vi "Build Tree.vi"(5 "Defer Updates (T)":bool=TRUE, 7 "Tree":refnum<vi>, 8 "error in":errorcluster, 11 "Tree Map in":refnum<class "Project Tree Map.lvclass">) -> (0 "error out":errorcluster, 3 "Tree Map out":refnum<class "Project Tree Map.lvclass">)   [LabVIEW 2020, in "VI Properties Editor.lvlib" / "Project Tree Map.lvclass"]
doc: "Builds the tree by adding the tree items one at a time."
uses:
  Project Tree Map.lvclass
  Project Tree Map.lvclass/Project Tree Map.ctl
  VI Properties Editor.lvlib
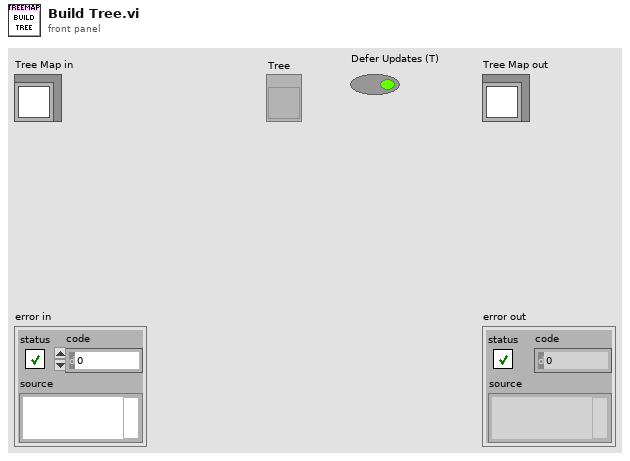
[diagram p1: front panel]
types:
  T1 = typedef "LVNodeAndColumnTypeDef.ctl" = cluster{"Node":string, "Column":i32}
  T2 = typedef "VI Properties Editor.lvlib/Project Tree Map.lvclass/Tree Key.ctl" = cluster{"Order":i32, "Hierarchy":string[]}
  T3 = typedef "VI Properties Editor.lvlib/Project Tree Map.lvclass/Tree Entry.ctl" = cluster{"Hierarchy":string[], "Name":string, "Columns":string[], "BG Color":u32, "Leaf":bool, "Symbol":string, "Parent Tag":string, "Order":i32, "Tag":string}
  T4 = typedef "imagedata.ctl" = cluster{"image type":i32, "image depth":i32, "image":u8[], "mask":u8[], "colors":u32[], "Rectangle":cluster{"left":i16, "top":i16, "right":i16, "bottom":i16}}
  T5 = map{string, cluster{"index":i32, "image data":T4}}
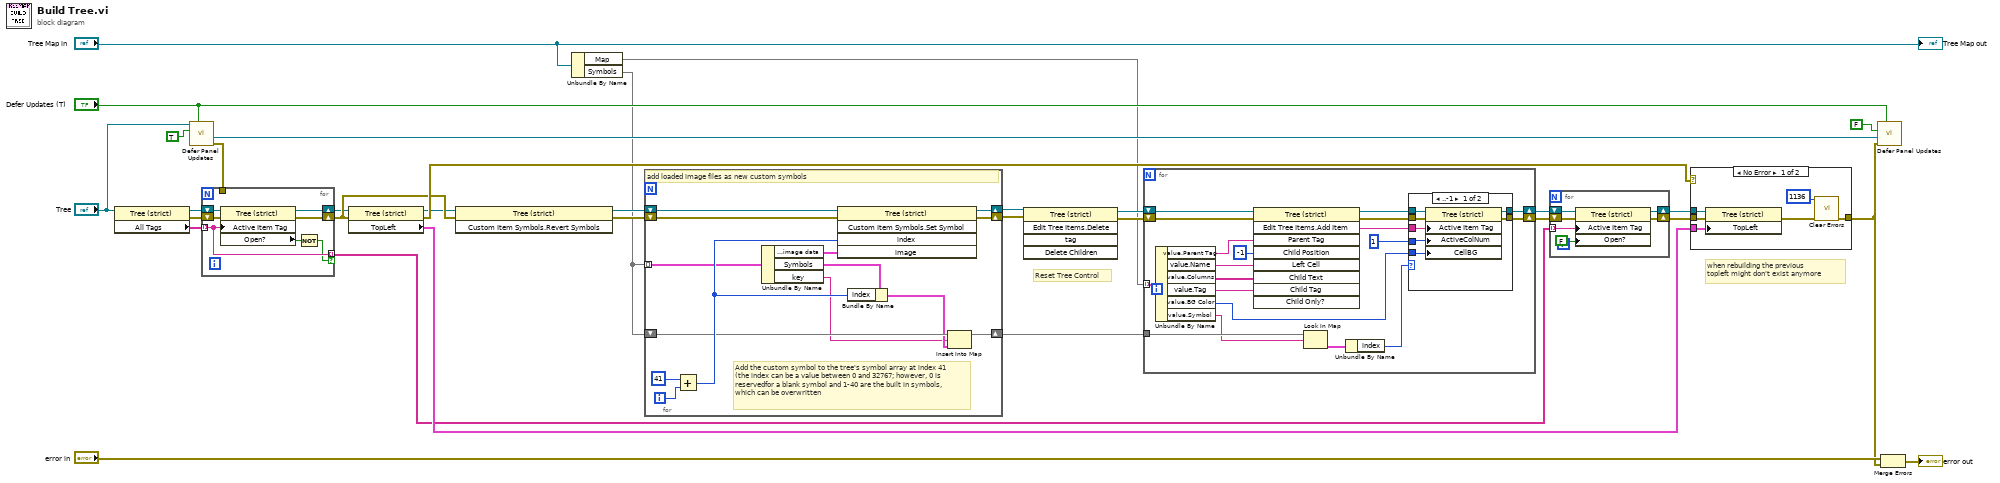
[diagram p0: block diagram]
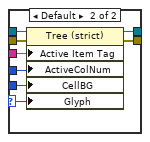
[diagram p2: hidden frame]
diagram:
  # "when rebuilding the previous\ntopleft might don't exist anymore"
  # "Reset Tree Control"
  n1 = property on="Property Node" class="Tree (strict)"(reference="Tree") -> (reference out=w17:refnum<vi>, error out=w29:errorcluster, "All Tags"=w18:string[])  [unwired: 1 in]
  n2 = call "Defer Panel Updates.vi"("Set Defer (T)"="Defer Updates (T)", "Defer"=TRUE, "Tree (Front Panel)"="Tree") -> ("error out"=w30:errorcluster, "Front Panel"=w9:refnum<vi>)  [unwired: 7 in]
  n3 = for {
    tunnel: w18 -> [w35] mode=indexing
    shift-right: [w33] -> w16
    shift-left: w17 -> [w37]
    tunnel: [w35] -> w15 mode=indexing if=w34
    tunnel: w30 -> [_]
    shift-right: [w38] -> w22
    shift-left: w29 -> [w39]
    n4 = property on="Property Node" class="Tree (strict)"(reference=w37, error in=w39, "Active Item Tag"=w35) -> (reference out=w33:refnum<vi>, error out=w38:errorcluster, "Open?"=w36:bool)
    n5 = Not(x=w36) -> (.not. x?=w34:bool)
  }
  n6 = property on="Property Node" class="Tree (strict)"(reference=w16, error in=w22) -> (reference out=w5:refnum<vi>, error out=w24:errorcluster, "TopLeft"=w19:T1)
  n7 = invoke on="Invoke Node" class="Tree (strict)" method="Custom Item Symbols.Revert Symbols"(reference=w5, error in=w22) -> (reference out=w4:refnum<vi>, error out=w23:errorcluster)  [unwired: 1 in, 1 out]
  n8 = Unbundle By Name("Tree Map in") -> ("Map"=w6:map{T2, T3}, "Symbols"=w3:T5)
  n9 = for {
    shift-right: [w49] -> w1
    shift-left: w4 -> [w50]
    shift-right: [w51] -> w21
    shift-left: w23 -> [w52]
    tunnel: w3 -> [w45] mode=indexing
    shift-right: [w43] -> w2
    shift-left: w3 -> [w44]
    i -> [w48]
    # "Add the custom symbol to the tree's symbol array at index 41 (the index can be a value between 0 and 32767; however, 0 is reservedfor a blank symbol and 1-40 are the built in symbols, which can be overwritten"
    # "add loaded image files as new custom symbols"
    n10 = Add(x=41 ("Index"), y=w48) -> (x+y=w53:i32)
    n11 = Unbundle By Name(w45) -> ("Symbols.image data"=w47:T4, "Symbols"=w41:cluster{"index":i32, "image data":T4}, "key"=w40:string)
    n12 = invoke on="Invoke Node" class="Tree (strict)" method="Custom Item Symbols.Set Symbol"(reference=w50, error in=w52, "index"=w53, "image"=w47) -> (reference out=w49:refnum<vi>, error out=w51:errorcluster)  [unwired: 1 in, 3 out]
    n13 = Bundle By Name(cluster=w41, "index"=w53) -> (w42:cluster{"index":i32, "image data":T4})
    n14 = Insert Into Map(map in=w44, key=w40, value=w42) -> (map out=w43:T5)  [unwired: 2 out]
  }
  n15 = invoke on="Invoke Node" class="Tree (strict)" method="Edit Tree Items.Delete"(reference=w1, error in=w21) -> (reference out=w20:refnum<vi>, error out=w32:errorcluster)  [unwired: 3 in, 3 out]
  n16 = for {
    shift-right: [w66] -> w13
    shift-left: w20 -> [w70]
    tunnel: w6 -> [w67] mode=indexing
    shift-right: [w71] -> w28
    shift-left: w32 -> [w72]
    tunnel: w2 -> [w65]
    n17 = Unbundle By Name(w67) -> ("value.Parent Tag"=w63:string, "value.Name"=w68:string, "value.Columns"=w69:string[], "value.Tag"=w62:string, "value.BG Color"=w64:u32, "value.Symbol"=w61:string)
    n18 = invoke on="Invoke Node" class="Tree (strict)" method="Edit Tree Items.Add Item"(reference=w70, error in=w72, "Parent Tag"=w63, "Child Position"=-1, "Left Cell"=w68, "Child Text"=w69, "Child Tag"=w62) -> (reference out=w59:refnum<vi>, error out=w60:errorcluster, "Edit Tree Items:Add Item"=w58:string)  [unwired: 2 in, 6 out]
    n19 = Look In Map(map=w65, key=w61) -> (value=w56:cluster{"index":i32, "image data":T4})  [unwired: 1 in, 1 out]
    n20 = Unbundle By Name(w56) -> ("index"=w55:i32)
    n21 = case shown="..-1" w55 {
      selector: w55 -> [_ w80]
      tunnel: w59 -> [w77 w85]
      tunnel: w60 -> [w79 w87]
      tunnel: w58 -> [w73 w84]
      tunnel: 1 ("Active Cell:Active Column Number") -> [w74 w83]
      tunnel: [w76 w82] -> w66
      tunnel: [w78 w86] -> w71
      tunnel: w64 -> [w75 w81]
      frame ..-1 {
        n22 = property on="Property Node" class="Tree (strict)"(reference=w77, error in=w79, "Active Item Tag"=w73, "ActiveColNum"=w74, "CellBG"=w75) -> (reference out=w76:refnum<vi>, error out=w78:errorcluster)
      }
      frame Default {
        n23 = property on="Property Node" class="Tree (strict)"(reference=w85, error in=w87, "Active Item Tag"=w84, "ActiveColNum"=w83, "CellBG"=w81, "Glyph"=w80) -> (reference out=w82:refnum<vi>, error out=w86:errorcluster)
      }
    }
  }
  n24 = for {
    shift-right: [w90] -> w14
    shift-left: w13 -> [w91]
    tunnel: w15 -> [w88] mode=indexing
    shift-right: [w92] -> w27
    shift-left: w28 -> [w93]
    n25 = property on="Property Node" class="Tree (strict)"(reference=w91, error in=w93, "Active Item Tag"=w88, "Open?"=FALSE ("Active Item:Open?")) -> (reference out=w90:refnum<vi>, error out=w92:errorcluster)
  }
  n26 = case shown="No Error" w24 {
    tunnel: w19 -> [w96 _]
    tunnel: w14 -> [w95 _]
    tunnel: w27 -> [w99 w100]
    tunnel: [w97 w100] -> w25
    frame No Error {
      n27 = property on="Property Node" class="Tree (strict)"(reference=w95, error in=w99, "TopLeft"=w96) -> (error out=w98:errorcluster)  [unwired: 1 out]
      n28 = call <vilib>:"Clear Errors.vi"("error in (no error)"=w98, "specific error code to clear (0: all)"=1136) -> ("error out"=w97:errorcluster)  [unwired: 4 in, 1 out]
    }
    frame Error {
    }
  }
  n29 = call "Defer Panel Updates.vi"("Set Defer (T)"="Defer Updates (T)", "error in (no error)"=w25, "Front Panel (Lookup)"=w9, "Defer"=FALSE ("Defer Panel Updates")) -> ()  [unwired: 6 in, 2 out]
  n30 = Merge Errors("error in", w25) -> (→"error out":errorcluster)
  "Tree Map out" <- "Tree Map in"
